vi "myRIO_BRig_RT_dataMTrig_CueLed_Tcycle.vi"() -> (2 "output_CueLed_Tcycle":i32)   [LabVIEW 2014]
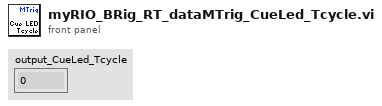
[diagram p1: front panel]
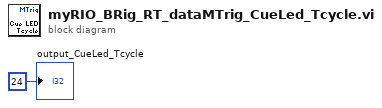
[diagram p0: block diagram]
diagram:
  "output_CueLed_Tcycle" <- 24 ("output_iBlock")
